vi "distance.vi"(1 "Point B":cluster{"X2":i32, "Y2":i32}, 2 "Point A":cluster{"X1":i32, "Y1":i32}) -> (0 "Distance":dbl)   [LabVIEW 2017]
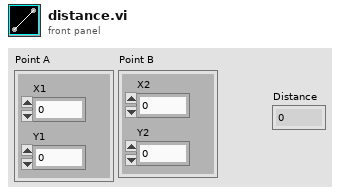
[diagram p1: front panel]
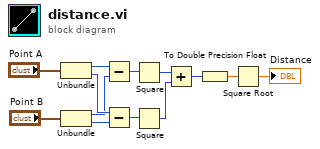
[diagram p0: block diagram]
diagram:
  n1 = Unbundle("Point A") -> ("X1"=w4:i32, "Y1"=w3:i32)
  n2 = Unbundle("Point B") -> ("X2"=w2:i32, "Y2"=w1:i32)
  n3 = Subtract(x=w4, y=w2) -> (x-y=w10:i32)
  n4 = Subtract(x=w3, y=w1) -> (x-y=w7:i32)
  n5 = Square(x=w10) -> (x^2=w9:i32)
  n6 = Square(x=w7) -> (x^2=w8:i32)
  n7 = Add(x=w9, y=w8) -> (x+y=w11:i32)
  n8 = To Double Precision Float(number=w11) -> (double precision float=w12:dbl)
  n9 = Square Root(x=w12) -> (sqrt(x)=→"Distance":dbl)
